vi "logStatusChecks.vi"(8 "error in (no error)":errorcluster, 10 "EventStatusChecks":T1, 11 "M1M3SAL in":refnum<class "M1M3SAL.lvclass">) -> (0 "error out":errorcluster, 3 "M1M3SAL out":refnum<class "M1M3SAL.lvclass">)   [LabVIEW 2016, in "M1M3SupportCommunicator.lvlib" / "M1M3SAL.lvclass"]
uses:
  M1M3SAL.lvclass
  DataTypes/Topics/EventStatusChecks.ctl
  DataTypes/Topics/Parts/Timestamp.ctl
  DataTypes/MessageHeader.ctl
  DataTypes/MessageTypes.ctl
  DataTypes/MessageTopics.ctl
  Common_RT_Utilities/U8ArrayBuilderAutoIndexing/U8ArrayBuilderAutoIndexing.lvclass
  M1M3SupportCommunicator.lvlib
  DataTypes/Topics/M1M3SupportTopics.lvlib
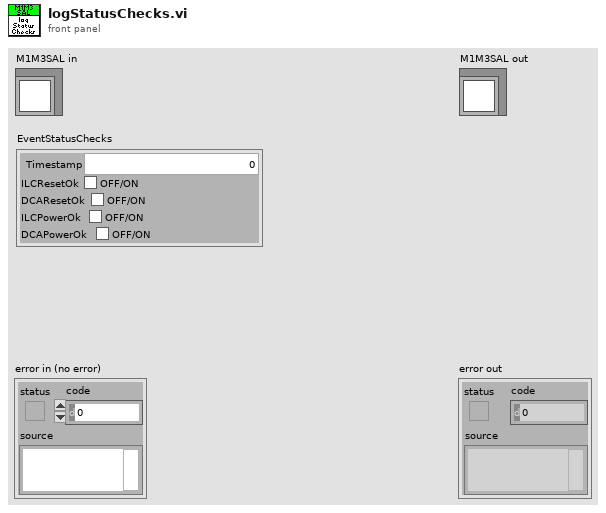
[diagram p1: front panel]
types:
  T1 = typedef "M1M3SupportTopics.lvlib/EventStatusChecks.ctl" = cluster{"Timestamp":T2, "ILCResetOk":bool, "DCAResetOk":bool, "ILCPowerOk":bool, "DCAPowerOk":bool}
  T2 = typedef "M1M3SupportTopics.lvlib/Timestamp.ctl" = dbl
  T3 = typedef "M1M3SupportCommunicator.lvlib/MessageHeader.ctl" = cluster{"Type":T4, "Topic":T5, "Size":i32}
  T4 = typedef "M1M3SupportCommunicator.lvlib/MessageTypes.ctl" = enum8{"None", "PutSample", "GetNextSample", "LogEvent", "GetEvent", "IssueCommand", "CommandId", "WaitForCompletion", "AcceptCommand", "AckCommand"}
  T5 = typedef "M1M3SupportCommunicator.lvlib/MessageTopics.ctl" = enum8{"None", "ForceActuatorData", "MirrorForceData", "HardpointData", "AirData", "DynamicData", "FPGAData", "IMSData", "ForceActuatorStatus", "ElevationData", "HardpointStatus", "HardpointActuatorChase", "AirStatus", "ForceActuatorSafetyChecks", "ForceActuatorTest", "ActuatorBroadcastCounter", "StatusChecks", "CellChecks", "HardpointActuatorBreakaway", "RaiseMirrorComplete", "ILCCommunication", "ElevationAngleChecks", "DetailedState", "ServoLoops", "ForceActuatorInfo", "LowerMirrorComplete", "HardpointActuatorInfo", "SettingsApplied", "ErrorCode", "StartupChecks", "SummaryState", "SettingVersions", "ActuatorTestStatus", "AppliedSettingsMatchStart", "Enable", "EnterMaintenance", "Standby", "AbortLowerM1M3", "ApplyAberrationByForces", "ApplyAOSCorrectionByBendingModes", "ClearAOSCorrection", "Start", "RaiseM1M3", "TestForceActuator", "LowerM1M3", "ApplyAOSCorrectionByForces", "Disable", "ApplyAberationByBendingMode", "TestHardpoint", "ManipulateM1M3", "ClearAberration", "Exit", "TestAir", "AbortRaiseM1M3", "MoveHardpointActuators", "ExitMaintenance", "Shutdown"}
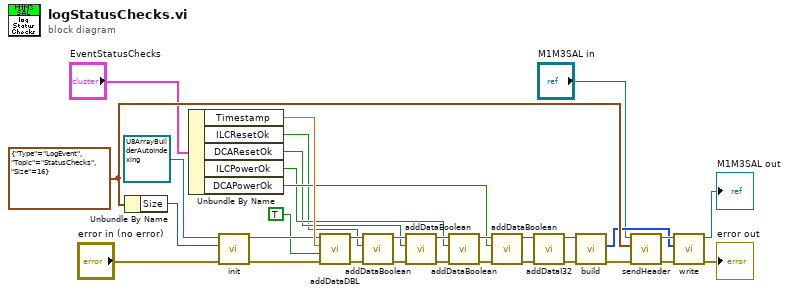
[diagram p0: block diagram]
diagram:
  w31 = T3 {"Type"=enum."LogEvent", "Topic"=enum."StatusChecks", "Size"=16} ("MessageHeader")
  n1 = Unbundle By Name(w31) -> ("Size"=w30:i32)
  n2 = Unbundle By Name("EventStatusChecks") -> ("Timestamp"=w21:T2, "ILCResetOk"=w6:bool, "DCAResetOk"=w7:bool, "ILCPowerOk"=w8:bool, "DCAPowerOk"=w9:bool)
  n3 = call "init.vi"("error in (no error)"="error in (no error)", "Size"=w30, "U8ArrayBuilderAutoIndexing in"=refnum<class "U8ArrayBuilderAutoIndexing.lvclass"> refnum ("RTUtilities.lvlib:U8ArrayBuilderAutoIndexing.lvclass")) -> ("error out"=w18:errorcluster, "U8ArrayBuilderAutoIndexing out"=w20:refnum<class "U8ArrayBuilderAutoIndexing.lvclass">)  [unwired: 7 in]
  n4 = call "addDataDBL.vi"("error in (no error)"=w18, "OverrideSwapBytes"=TRUE, "Data"=w21, "U8ArrayBuilderAutoIndexing in"=w20) -> ("error out"=w12:errorcluster, "U8ArrayBuilderAutoIndexing out"=w13:refnum<class "U8ArrayBuilderAutoIndexing.lvclass">)  [unwired: 6 in]
  n5 = call "addDataBoolean.vi"("error in (no error)"=w12, "Data"=w6, "U8ArrayBuilderAutoIndexing in"=w13) -> ("error out"=w17:errorcluster, "U8ArrayBuilderAutoIndexing out"=w16:refnum<class "U8ArrayBuilderAutoIndexing.lvclass">)  [unwired: 7 in]
  n6 = call "addDataBoolean.vi"("error in (no error)"=w17, "Data"=w7, "U8ArrayBuilderAutoIndexing in"=w16) -> ("error out"=w15:errorcluster, "U8ArrayBuilderAutoIndexing out"=w14:refnum<class "U8ArrayBuilderAutoIndexing.lvclass">)  [unwired: 7 in]
  n7 = call "addDataBoolean.vi"("error in (no error)"=w15, "Data"=w8, "U8ArrayBuilderAutoIndexing in"=w14) -> ("error out"=w11:errorcluster, "U8ArrayBuilderAutoIndexing out"=w10:refnum<class "U8ArrayBuilderAutoIndexing.lvclass">)  [unwired: 7 in]
  n8 = call "addDataBoolean.vi"("error in (no error)"=w11, "Data"=w9, "U8ArrayBuilderAutoIndexing in"=w10) -> ("error out"=w2:errorcluster, "U8ArrayBuilderAutoIndexing out"=w4:refnum<class "U8ArrayBuilderAutoIndexing.lvclass">)  [unwired: 7 in]
  n9 = call "addDataI32.vi"("error in (no error)"=w2, "U8ArrayBuilderAutoIndexing in"=w4) -> ("error out"=w1:errorcluster, "U8ArrayBuilderAutoIndexing out"=w3:refnum<class "U8ArrayBuilderAutoIndexing.lvclass">)  [unwired: 8 in]
  n10 = call "build.vi"("error in (no error)"=w1, "U8ArrayBuilderAutoIndexing in"=w3) -> ("error out"=w27:errorcluster, "Array"=w28:u8[])  [unwired: 7 in, 1 out]
  n11 = call "sendHeader.vi"("error in (no error)"=w27, "MessageHeader"=w31, "M1M3SAL in"="M1M3SAL in") -> ("error out"=w26:errorcluster, "M1M3SAL out"=w29:refnum<class "M1M3SAL.lvclass">)  [unwired: 7 in]
  n12 = call "write.vi"("error in (no error)"=w26, "Data"=w28, "M1M3SAL in"=w29) -> ("error out"=→"error out":errorcluster, "M1M3SAL out"=→"M1M3SAL out":refnum<class "M1M3SAL.lvclass">)  [unwired: 7 in]
